vi "GUI_StagingEnergyCalib.vi"() -> ()   [LabVIEW 2013]
uses:
  Device Driver/StagingAnalysis/SubVis/SubVi/polTypDef.ctl
  Device Driver/StagingAnalysis/SubVis/energyCalibTypdef.ctl
  shared programs/GUI_Template/GUI_master/tcp new data cluster.ctl
  <vilib>/Analysis/1siggen.llb/Ramp Pattern by Samples.vi
  Device Driver/BaseDriver/BaseDriver.lvclass
  <vilib>/Analysis/NI_AALBase.lvlib
panel:
  out "Ramp Pattern":dbl[](graph)=[0.0, 4.5045045045045005e-06, 9.009009009009001e-06, 1.3513513513513502e-05, 1.8018018018018002e-05, 2.2522522522522503e-05, 2.7027027027027003e-05, 3.1531531531531504e-05, 3.6036036036036004e-05, 4.0540540540540505e-05, 4.5045045045045005e-05, 4.9549549549549506e-05, 5.4054054054054006e-05, 5.8558558558558507e-05, 6.306306306306301e-05, 6.756756756756751e-05, 7.207207207207201e-05, 7.657657657657652e-05, 8.108108108108101e-05, 8.558558558558552e-05, 9.009009009009001e-05, 9.459459459459452e-05, 9.909909909909901e-05, 0.00010360360360360352, 0.00010810810810810801, 0.00011261261261261252, 0.00011711711711711701, 0.00012162162162162152, 0.00012612612612612601, 0.00013063063063063052, 0.00013513513513513503, 0.0001396396396396395, 0.00014414414414414402, 0.00014864864864864852, 0.00015315315315315303, 0.0001576576576576575, 0.00016216216216216202, 0.00016666666666666653, 0.00017117117117117103, 0.00017567567567567554, 0.00018018018018018002, 0.00018468468468468453, 0.00018918918918918903, 0.00019369369369369354, 0.00019819819819819802, 0.00020270270270270253, 0.00020720720720720704, 0.00021171171171171154, 0.00021621621621621602, 0.00022072072072072053, 0.00022522522522522504, 0.00022972972972972955, 0.00023423423423423403, 0.00023873873873873853, 0.00024324324324324304, 0.00024774774774774755, 0.00025225225225225203, 0.00025675675675675656, 0.00026126126126126104, 0.0002657657657657655, 0.00027027027027027006, 0.00027477477477477454, 0.000279279279279279, 0.00028378378378378355, 0.00028828828828828803, 0.00029279279279279257, 0.00029729729729729705, 0.00030180180180180153, 0.00030630630630630606, 0.00031081081081081054, 0.000315315315315315, 0.00031981981981981956, 0.00032432432432432404, 0.00032882882882882857, 0.00033333333333333305, 0.00033783783783783753, 0.00034234234234234207, 0.00034684684684684655, 0.0003513513513513511, 0.00035585585585585556, 0.00036036036036036004, 0.0003648648648648646, 0.00036936936936936906, 0.00037387387387387354, 0.00037837837837837807, 0.00038288288288288255, 0.0003873873873873871, 0.00039189189189189156, 0.00039639639639639604, 0.0004009009009009006, 0.00040540540540540506, 0.00040990990990990954, 0.0004144144144144141, 0.00041891891891891855, 0.0004234234234234231, 0.00042792792792792757, 0.00043243243243243205, 0.0004369369369369366, 0.00044144144144144106, 0.00044594594594594554, 0.0004504504504504501, 0.00045495495495495456, 0.0004594594594594591, 0.00046396396396396357, 0.00046846846846846805, 0.0004729729729729726, 0.00047747747747747707, 0.00048198198198198155, 0.0004864864864864861, 0.0004909909909909906, 0.0004954954954954951, 0.0004999999999999996, 0.0005045045045045041, 0.0005090090090090085, 0.0005135135135135131, 0.0005180180180180176, 0.0005225225225225221, 0.0005270270270270266, 0.000531531531531531, 0.0005360360360360356, 0.0005405405405405401, 0.0005450450450450446, 0.0005495495495495491, 0.0005540540540540536, 0.000558558558558558, 0.0005630630630630626, 0.0005675675675675671, 0.0005720720720720716, 0.0005765765765765761, 0.0005810810810810805, 0.0005855855855855851, 0.0005900900900900896, 0.0005945945945945941, 0.0005990990990990986, 0.0006036036036036031, 0.0006081081081081076, 0.0006126126126126121, 0.0006171171171171166, 0.0006216216216216211, 0.0006261261261261256, 0.00063063063063063, 0.0006351351351351346, 0.0006396396396396391, 0.0006441441441441436, 0.0006486486486486481, 0.0006531531531531526, 0.0006576576576576571, 0.0006621621621621616, 0.0006666666666666661, 0.0006711711711711706, 0.0006756756756756751, 0.0006801801801801797, 0.0006846846846846841, 0.0006891891891891886, 0.0006936936936936931, 0.0006981981981981976, 0.0007027027027027022, 0.0007072072072072066, 0.0007117117117117111, 0.0007162162162162156, 0.0007207207207207201, 0.0007252252252252246, 0.0007297297297297292, 0.0007342342342342336, 0.0007387387387387381, 0.0007432432432432426, 0.0007477477477477471, 0.0007522522522522517, 0.0007567567567567561, 0.0007612612612612606, 0.0007657657657657651, 0.0007702702702702696, 0.0007747747747747742, 0.0007792792792792786, 0.0007837837837837831, 0.0007882882882882876, 0.0007927927927927921, 0.0007972972972972966, 0.0008018018018018012, 0.0008063063063063056, 0.0008108108108108101, 0.0008153153153153146, 0.0008198198198198191, 0.0008243243243243237, 0.0008288288288288281, 0.0008333333333333326, 0.0008378378378378371, 0.0008423423423423416, 0.0008468468468468462, 0.0008513513513513507, 0.0008558558558558551, 0.0008603603603603596, 0.0008648648648648641, 0.0008693693693693687, 0.0008738738738738732, 0.0008783783783783776, 0.0008828828828828821, 0.0008873873873873866, 0.0008918918918918911, 0.0008963963963963957, 0.0009009009009009002, 0.0009054054054054046, 0.0009099099099099091, 0.0009144144144144136, 0.0009189189189189182, 0.0009234234234234227, 0.0009279279279279271, 0.0009324324324324316, 0.0009369369369369361, 0.0009414414414414407, 0.0009459459459459452, 0.0009504504504504497, 0.0009549549549549541, 0.0009594594594594586, 0.0009639639639639631, 0.0009684684684684677, 0.0009729729729729722, 0.0009774774774774766, 0.0009819819819819812, 0.0009864864864864856, 0.0009909909909909902, 0.0009954954954954946, 0.0009999999999999992, 0.0010045045045045037, 0.0010090090090090081, 0.0010135135135135127, 0.001018018018018017, 0.0010225225225225217, 0.0010270270270270263, 0.0010315315315315306, 0.0010360360360360352, 0.0010405405405405396, 0.0010450450450450442, 0.0010495495495495488, 0.0010540540540540531, 0.0010585585585585577, 0.001063063063063062, 0.0010675675675675667, 0.0010720720720720713, 0.0010765765765765756, 0.0010810810810810802, 0.0010855855855855846, 0.0010900900900900892, 0.0010945945945945936, 0.0010990990990990982, 0.0011036036036036027, 0.0011081081081081071, 0.0011126126126126117, 0.001117117117117116, 0.0011216216216216207, 0.0011261261261261252, 0.0011306306306306296, 0.0011351351351351342, 0.0011396396396396386, 0.0011441441441441432, 0.0011486486486486478, 0.0011531531531531521, 0.0011576576576576567, 0.001162162162162161, 0.0011666666666666657, 0.0011711711711711703, 0.0011756756756756746, 0.0011801801801801792, 0.0011846846846846836, 0.0011891891891891882, 0.0011936936936936928, 0.0011981981981981971, 0.0012027027027027017, 0.0012072072072072061, 0.0012117117117117107, 0.0012162162162162153, 0.0012207207207207197, 0.0012252252252252242, 0.0012297297297297286, 0.0012342342342342332, 0.0012387387387387378, 0.0012432432432432422, 0.0012477477477477468, 0.0012522522522522511, 0.0012567567567567557, 0.00126126126126126, 0.0012657657657657647, 0.0012702702702702693, 0.0012747747747747736, 0.0012792792792792782, 0.0012837837837837826, 0.0012882882882882872, 0.0012927927927927918, 0.0012972972972972961, 0.0013018018018018007, 0.001306306306306305, 0.0013108108108108097, 0.0013153153153153143, 0.0013198198198198187, 0.0013243243243243232, 0.0013288288288288276, 0.0013333333333333322, 0.0013378378378378368, 0.0013423423423423412, 0.0013468468468468458, 0.0013513513513513501, 0.0013558558558558547, 0.0013603603603603593, 0.0013648648648648637, 0.0013693693693693683, 0.0013738738738738726, 0.0013783783783783772, 0.0013828828828828818, 0.0013873873873873862, 0.0013918918918918908, 0.0013963963963963951, 0.0014009009009008997, 0.0014054054054054043, 0.0014099099099099087, 0.0014144144144144133, 0.0014189189189189177, 0.0014234234234234222, 0.0014279279279279266, 0.0014324324324324312, 0.0014369369369369358, 0.0014414414414414402, 0.0014459459459459448, 0.0014504504504504491, 0.0014549549549549537, 0.0014594594594594583, 0.0014639639639639627, 0.0014684684684684673, 0.0014729729729729716, 0.0014774774774774762, 0.0014819819819819808, 0.0014864864864864852, 0.0014909909909909898, 0.0014954954954954941, 0.0014999999999999987, 0.0015045045045045033, 0.0015090090090090077, 0.0015135135135135123, 0.0015180180180180167, 0.0015225225225225212, 0.0015270270270270258, 0.0015315315315315302, 0.0015360360360360348, 0.0015405405405405392, 0.0015450450450450437, 0.0015495495495495483, 0.0015540540540540527, 0.0015585585585585573, 0.0015630630630630617, 0.0015675675675675663, 0.0015720720720720708, 0.0015765765765765752, 0.0015810810810810798, 0.0015855855855855842, 0.0015900900900900888, 0.0015945945945945931, 0.0015990990990990977, 0.0016036036036036023, 0.0016081081081081067, 0.0016126126126126113, 0.0016171171171171156, 0.0016216216216216202, 0.0016261261261261248, 0.0016306306306306292, 0.0016351351351351338, 0.0016396396396396382, 0.0016441441441441427, 0.0016486486486486473, 0.0016531531531531517, 0.0016576576576576563, 0.0016621621621621607, 0.0016666666666666653, 0.0016711711711711698, 0.0016756756756756742, 0.0016801801801801788, 0.0016846846846846832, 0.0016891891891891878, 0.0016936936936936924, 0.0016981981981981967, 0.0017027027027027013, 0.0017072072072072057, 0.0017117117117117103, 0.0017162162162162149, 0.0017207207207207192, 0.0017252252252252238, 0.0017297297297297282, 0.0017342342342342328, 0.0017387387387387374, 0.0017432432432432417, 0.0017477477477477463, 0.0017522522522522507, 0.0017567567567567553, 0.0017612612612612597, 0.0017657657657657643, 0.0017702702702702688, 0.0017747747747747732, 0.0017792792792792778, 0.0017837837837837822, 0.0017882882882882868, 0.0017927927927927914, 0.0017972972972972957, 0.0018018018018018003, 0.0018063063063063047, 0.0018108108108108093, 0.0018153153153153139, 0.0018198198198198182, 0.0018243243243243228, 0.0018288288288288272, 0.0018333333333333318, 0.0018378378378378364, 0.0018423423423423407, 0.0018468468468468453, 0.0018513513513513497, 0.0018558558558558543, 0.0018603603603603589, 0.0018648648648648633, 0.0018693693693693678, 0.0018738738738738722, 0.0018783783783783768, 0.0018828828828828814, 0.0018873873873873858, 0.0018918918918918903, 0.0018963963963963947, 0.0019009009009008993, 0.001905405405405404, 0.0019099099099099083, 0.0019144144144144129, 0.0019189189189189172, 0.0019234234234234218, 0.0019279279279279262, 0.0019324324324324308, 0.0019369369369369354, 0.0019414414414414397, 0.0019459459459459443, 0.0019504504504504487, 0.0019549549549549533, 0.0019594594594594577, 0.0019639639639639625, 0.001968468468468467, 0.001972972972972971, 0.001977477477477476, 0.0019819819819819804, 0.0019864864864864848, 0.001990990990990989, 0.001995495495495494, 0.0019999999999999983, 0.0020045045045045027, 0.0020090090090090075, 0.002013513513513512, 0.0020180180180180162, 0.0020225225225225206, 0.0020270270270270254, 0.0020315315315315298, 0.002036036036036034, 0.002040540540540539, 0.0020450450450450433, 0.0020495495495495477, 0.0020540540540540525, 0.002058558558558557, 0.0020630630630630612, 0.0020675675675675656, 0.0020720720720720704, 0.002076576576576575, 0.002081081081081079, 0.002085585585585584, 0.0020900900900900883, 0.0020945945945945927, 0.0020990990990990975, 0.002103603603603602, 0.0021081081081081063, 0.0021126126126126106, 0.0021171171171171154, 0.00212162162162162, 0.002126126126126124, 0.002130630630630629, 0.0021351351351351334, 0.0021396396396396377, 0.0021441441441441425, 0.002148648648648647, 0.0021531531531531513, 0.0021576576576576557, 0.0021621621621621605, 0.002166666666666665, 0.002171171171171169, 0.002175675675675674, 0.0021801801801801784, 0.0021846846846846828, 0.002189189189189187, 0.002193693693693692, 0.0021981981981981963, 0.0022027027027027007, 0.0022072072072072055, 0.00221171171171171, 0.0022162162162162142, 0.002220720720720719, 0.0022252252252252234, 0.0022297297297297278, 0.002234234234234232, 0.002238738738738737, 0.0022432432432432413, 0.0022477477477477457, 0.0022522522522522505, 0.002256756756756755, 0.0022612612612612592, 0.002265765765765764, 0.0022702702702702684, 0.002274774774774773, 0.002279279279279277, 0.002283783783783782, 0.0022882882882882863, 0.0022927927927927907, 0.0022972972972972955, 0.0023018018018018, 0.0023063063063063043, 0.002310810810810809, 0.0023153153153153134, 0.002319819819819818, 0.002324324324324322, 0.002328828828828827, 0.0023333333333333314, 0.0023378378378378357, 0.0023423423423423405, 0.002346846846846845, 0.0023513513513513493, 0.0023558558558558537, 0.0023603603603603585, 0.002364864864864863, 0.002369369369369367, 0.002373873873873872, 0.0023783783783783764, 0.0023828828828828807, 0.0023873873873873856, 0.00239189189189189, 0.0023963963963963943, 0.0024009009009008987, 0.0024054054054054035, 0.002409909909909908, 0.0024144144144144122, 0.002418918918918917, 0.0024234234234234214, 0.0024279279279279258, 0.0024324324324324306, 0.002436936936936935, 0.0024414414414414393, 0.0024459459459459437, 0.0024504504504504485, 0.002454954954954953, 0.0024594594594594572, 0.002463963963963962, 0.0024684684684684664, 0.002472972972972971, 0.0024774774774774756, 0.00248198198198198, 0.0024864864864864843, 0.0024909909909909887, 0.0024954954954954935, 0.002499999999999998, 0.0025045045045045023, 0.002509009009009007, 0.0025135135135135114, 0.002518018018018016, 0.00252252252252252, 0.002527027027027025, 0.0025315315315315294, 0.0025360360360360337, 0.0025405405405405385, 0.002545045045045043, 0.0025495495495495473, 0.002554054054054052, 0.0025585585585585565, 0.002563063063063061, 0.002567567567567565, 0.00257207207207207, 0.0025765765765765744, 0.0025810810810810787, 0.0025855855855855835, 0.002590090090090088, 0.0025945945945945923, 0.002599099099099097, 0.0026036036036036015, 0.002608108108108106, 0.00261261261261261, 0.002617117117117115, 0.0026216216216216194, 0.0026261261261261238, 0.0026306306306306286, 0.002635135135135133, 0.0026396396396396373, 0.002644144144144142, 0.0026486486486486465, 0.002653153153153151, 0.0026576576576576552, 0.00266216216216216, 0.0026666666666666644, 0.0026711711711711688, 0.0026756756756756736, 0.002680180180180178, 0.0026846846846846823, 0.0026891891891891867, 0.0026936936936936915, 0.002698198198198196, 0.0027027027027027003, 0.002707207207207205, 0.0027117117117117094, 0.002716216216216214, 0.0027207207207207186, 0.002725225225225223, 0.0027297297297297273, 0.0027342342342342317, 0.0027387387387387365, 0.002743243243243241, 0.0027477477477477453, 0.00275225225225225, 0.0027567567567567544, 0.002761261261261259, 0.0027657657657657636, 0.002770270270270268, 0.0027747747747747724, 0.0027792792792792767, 0.0027837837837837815, 0.002788288288288286, 0.0027927927927927903, 0.002797297297297295, 0.0028018018018017995, 0.002806306306306304, 0.0028108108108108086, 0.002815315315315313, 0.0028198198198198174, 0.0028243243243243218, 0.0028288288288288266, 0.002833333333333331, 0.0028378378378378353, 0.00284234234234234, 0.0028468468468468445, 0.002851351351351349, 0.0028558558558558532, 0.002860360360360358, 0.0028648648648648624, 0.0028693693693693668, 0.0028738738738738716, 0.002878378378378376, 0.0028828828828828803, 0.002887387387387385, 0.0028918918918918895, 0.002896396396396394, 0.0029009009009008982, 0.002905405405405403, 0.0029099099099099074, 0.002914414414414412, 0.0029189189189189166, 0.002923423423423421, 0.0029279279279279253, 0.00293243243243243, 0.0029369369369369345, 0.002941441441441439, 0.0029459459459459433, 0.002950450450450448, 0.0029549549549549524, 0.002959459459459457, 0.0029639639639639616, 0.002968468468468466, 0.0029729729729729704, 0.002977477477477475, 0.0029819819819819795, 0.002986486486486484, 0.0029909909909909883, 0.002995495495495493, 0.0029999999999999975, 0.003004504504504502, 0.0030090090090090066, 0.003013513513513511, 0.0030180180180180154, 0.0030225225225225198, 0.0030270270270270246, 0.003031531531531529, 0.0030360360360360333, 0.003040540540540538, 0.0030450450450450425, 0.003049549549549547, 0.0030540540540540517, 0.003058558558558556, 0.0030630630630630604, 0.0030675675675675648, 0.0030720720720720696, 0.003076576576576574, 0.0030810810810810783, 0.003085585585585583, 0.0030900900900900875, 0.003094594594594592, 0.0030990990990990967, 0.003103603603603601, 0.0031081081081081054, 0.00311261261261261, 0.0031171171171171146, 0.003121621621621619, 0.0031261261261261233, 0.003130630630630628, 0.0031351351351351325, 0.003139639639639637, 0.0031441441441441417, 0.003148648648648646, 0.0031531531531531504, 0.003157657657657655, 0.0031621621621621596, 0.003166666666666664, 0.0031711711711711684, 0.003175675675675673, 0.0031801801801801775, 0.003184684684684682, 0.0031891891891891863, 0.003193693693693691, 0.0031981981981981955, 0.0032027027027027, 0.0032072072072072046, 0.003211711711711709, 0.0032162162162162134, 0.003220720720720718, 0.0032252252252252226, 0.003229729729729727, 0.0032342342342342313, 0.003238738738738736, 0.0032432432432432405, 0.003247747747747745, 0.0032522522522522497, 0.003256756756756754, 0.0032612612612612584, 0.003265765765765763, 0.0032702702702702676, 0.003274774774774772, 0.0032792792792792763, 0.003283783783783781, 0.0032882882882882855, 0.00329279279279279, 0.0032972972972972947, 0.003301801801801799, 0.0033063063063063034, 0.0033108108108108082, 0.0033153153153153126, 0.003319819819819817, 0.0033243243243243213, 0.003328828828828826, 0.0033333333333333305, 0.003337837837837835, 0.0033423423423423397, 0.003346846846846844, 0.0033513513513513484, 0.003355855855855853, 0.0033603603603603576, 0.003364864864864862, 0.0033693693693693664, 0.003373873873873871, 0.0033783783783783755, 0.00338288288288288, 0.0033873873873873847, 0.003391891891891889, 0.0033963963963963935, 0.003400900900900898, 0.0034054054054054026, 0.003409909909909907, 0.0034144144144144114, 0.003418918918918916, 0.0034234234234234205, 0.003427927927927925, 0.0034324324324324297, 0.003436936936936934, 0.0034414414414414385, 0.003445945945945943, 0.0034504504504504476, 0.003454954954954952, 0.0034594594594594564, 0.003463963963963961, 0.0034684684684684656, 0.00347297297297297, 0.0034774774774774747, 0.003481981981981979, 0.0034864864864864835, 0.003490990990990988, 0.0034954954954954927, 0.003499999999999997, 0.0035045045045045014, 0.003509009009009006, 0.0035135135135135106, 0.003518018018018015, 0.0035225225225225193, 0.003527027027027024, 0.0035315315315315285, 0.003536036036036033, 0.0035405405405405377, 0.003545045045045042, 0.0035495495495495464, 0.0035540540540540512, 0.0035585585585585556, 0.00356306306306306, 0.0035675675675675643, 0.003572072072072069, 0.0035765765765765735, 0.003581081081081078, 0.0035855855855855827, 0.003590090090090087, 0.0035945945945945914, 0.0035990990990990963, 0.0036036036036036006, 0.003608108108108105, 0.0036126126126126094, 0.003617117117117114, 0.0036216216216216185, 0.003626126126126123, 0.0036306306306306277, 0.003635135135135132, 0.0036396396396396365, 0.0036441441441441413, 0.0036486486486486456, 0.00365315315315315, 0.0036576576576576544, 0.003662162162162159, 0.0036666666666666636, 0.003671171171171168, 0.0036756756756756727, 0.003680180180180177, 0.0036846846846846815, 0.003689189189189186, 0.0036936936936936907, 0.003698198198198195, 0.0037027027027026994, 0.003707207207207204, 0.0037117117117117086, 0.003716216216216213, 0.0037207207207207178, 0.003725225225225222, 0.0037297297297297265, 0.003734234234234231, 0.0037387387387387357, 0.00374324324324324, 0.0037477477477477444, 0.0037522522522522492, 0.0037567567567567536, 0.003761261261261258, 0.0037657657657657628, 0.003770270270270267, 0.0037747747747747715, 0.003779279279279276, 0.0037837837837837807, 0.003788288288288285, 0.0037927927927927894, 0.0037972972972972942, 0.0038018018018017986, 0.003806306306306303, 0.003810810810810808, 0.003815315315315312, 0.0038198198198198165, 0.003824324324324321, 0.0038288288288288257, 0.00383333333333333, 0.0038378378378378345, 0.0038423423423423393, 0.0038468468468468436, 0.003851351351351348, 0.0038558558558558524, 0.003860360360360357, 0.0038648648648648616, 0.003869369369369366, 0.0038738738738738707, 0.003878378378378375, 0.0038828828828828795, 0.0038873873873873843, 0.0038918918918918887, 0.003896396396396393, 0.0039009009009008974, 0.003905405405405402, 0.003909909909909907, 0.003914414414414411, 0.003918918918918915, 0.00392342342342342, 0.003927927927927925, 0.003932432432432429, 0.003936936936936934, 0.0039414414414414385, 0.003945945945945942, 0.003950450450450447, 0.003954954954954952, 0.003959459459459456, 0.003963963963963961, 0.003968468468468465, 0.0039729729729729695, 0.003977477477477474, 0.003981981981981978, 0.003986486486486483, 0.003990990990990988, 0.003995495495495492, 0.003999999999999997, 0.004004504504504501, 0.004009009009009005, 0.00401351351351351, 0.004018018018018015, 0.004022522522522519, 0.004027027027027024, 0.0040315315315315285, 0.0040360360360360325, 0.004040540540540537, 0.004045045045045041, 0.004049549549549546, 0.004054054054054051, 0.004058558558558555, 0.0040630630630630596, 0.004067567567567564, 0.004072072072072068, 0.004076576576576573, 0.004081081081081078, 0.004085585585585582, 0.004090090090090087, 0.0040945945945945915, 0.004099099099099095, 0.0041036036036036, 0.004108108108108105, 0.004112612612612609, 0.004117117117117114, 0.0041216216216216186, 0.0041261261261261225, 0.004130630630630627, 0.004135135135135131, 0.004139639639639636, 0.004144144144144141, 0.004148648648648645, 0.00415315315315315, 0.004157657657657654, 0.004162162162162158, 0.004166666666666663, 0.004171171171171168, 0.004175675675675672, 0.004180180180180177, 0.0041846846846846815, 0.004189189189189185, 0.00419369369369369, 0.004198198198198195, 0.004202702702702699, 0.004207207207207204, 0.004211711711711708, 0.0042162162162162125, 0.004220720720720717, 0.004225225225225221, 0.004229729729729726, 0.004234234234234231, 0.004238738738738735, 0.00424324324324324, 0.004247747747747744, 0.004252252252252248, 0.004256756756756753, 0.004261261261261258, 0.004265765765765762, 0.004270270270270267, 0.0042747747747747715, 0.0042792792792792755, 0.00428378378378378, 0.004288288288288285, 0.004292792792792789, 0.004297297297297294, 0.004301801801801798, 0.004306306306306303, 0.004310810810810807, 0.004315315315315311, 0.004319819819819816, 0.004324324324324321, 0.004328828828828825, 0.00433333333333333, 0.0043378378378378345, 0.004342342342342338, 0.004346846846846843, 0.004351351351351348, 0.004355855855855852, 0.004360360360360357, 0.004364864864864862, 0.0043693693693693655, 0.00437387387387387, 0.004378378378378374, 0.004382882882882879, 0.004387387387387384, 0.004391891891891888, 0.004396396396396393, 0.004400900900900897, 0.004405405405405401, 0.004409909909909906, 0.004414414414414411, 0.004418918918918915, 0.00442342342342342, 0.0044279279279279245, 0.0044324324324324284, 0.004436936936936933, 0.004441441441441438, 0.004445945945945942, 0.004450450450450447, 0.004454954954954952, 0.0044594594594594555, 0.00446396396396396, 0.004468468468468464, 0.004472972972972969, 0.004477477477477474, 0.004481981981981978, 0.004486486486486483, 0.0044909909909909874, 0.004495495495495491, 0.004499999999999996]
  in  "end":dbl=0.004499999999999996
  in  "file path (dialog if empty)":path=path "V:/Y2013/02-Feb/13_0207/analysis/s8.txt"
  in  "load":bool=TRUE
  in  "startlinear":dbl=0.000828
  out "x+1":dbl=188.0
  in  "old calib":bool=TRUE
  in  "take data":bool
  out "energyCalib":T1={"p-pol"={"Beam1"=0.585575, "Beam2"=0.414425, "Tele"=0.004938, "startLinear"=0.0007, "best fit parameters"={"0"=0.88643, "1"=-3261.333361, "2"=6330262.535463, "3"=-3978154912.425541}}, "s-pol"={"Beam1"=0.585575, "Beam2"=0.414424708329109, "Tele"=0.004938, "position for fit"=0.000828, "best fit parameters"={"0"=0.042645, "1"=208.033972, "2"=-303343.534936, "3"=170108367.568354}}, "B-CaveFilter"=0.165}
  in  "toDB":bool=TRUE
  in  "B-Cave-Filter (value)":dbl=0.165
  in  "BCaveFilterStatus":enum16{"B-Cave filter in", "B-Cave filter out"}(ring)=enum."B-Cave filter out"
  in  "Polarization":T2=enum."s-polarized"
  in  "fit":bool
  in  "reset":bool
  out "XY Graph":cluster{dbl[], dbl[]}[](graph)
  out "GUIdevice 1":string="StagingPXISlow"
  in  "Measurements.Analysis2::1":dbl=6.4710866e-05 caption="Energy in raw" min=0.0 max=0.0
  in  "Measurements.Analysis1::1":dbl=3.059521e-06 caption="Energy out raw" min=0.0 max=0.0
  out "device status::1":string="no scan"
  in  "stop":bool
  out "UDP error message":string
  in  "insert tag":bool=TRUE
  # "last calib:"
  # "V:\\Y2012\\12-Dec\\12_1213\\analysis\\s4.txt"
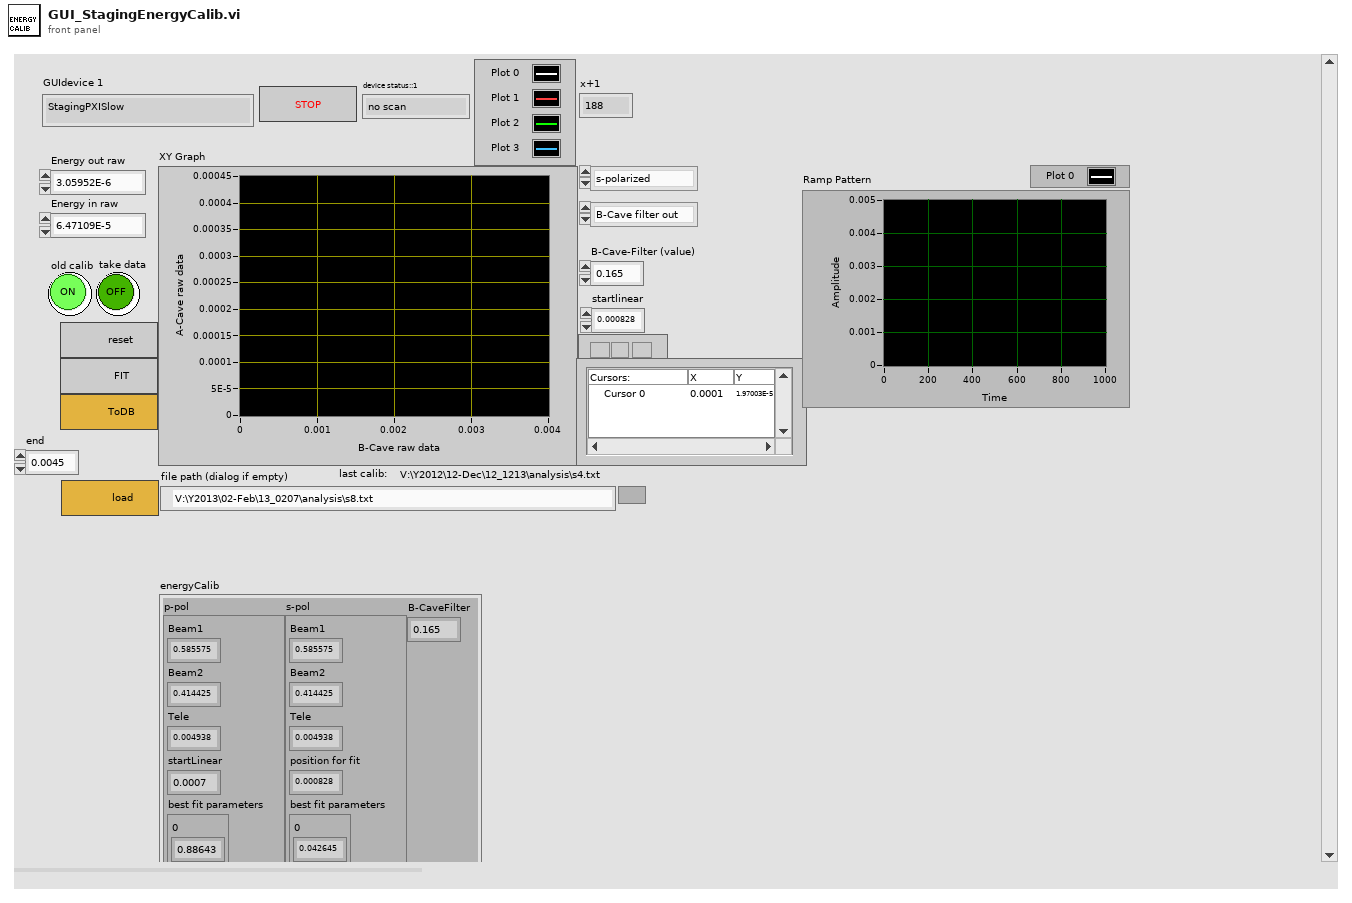
[diagram p1: front panel]
types:
  T1 = typedef "energyCalibTypdef.ctl" = cluster{"p-pol":cluster{"Beam1":dbl, "Beam2":dbl, "Tele":dbl, "startLinear":dbl, "best fit parameters":cluster{"0":dbl, "1":dbl, "2":dbl, "3":dbl}}, "s-pol":cluster{"Beam1":dbl, "Beam2":dbl, "Tele":dbl, "position for fit":dbl, "best fit parameters":cluster{"0":dbl, "1":dbl, "2":dbl, "3":dbl}}, "B-CaveFilter":dbl}
  T2 = typedef "polTypDef.ctl" = enum16{"p-polarized", "s-polarized"}
  T3 = typedef "tcp new data cluster.ctl" = cluster{"EventEnum":enum16{"new data", "connection status update"}, "Device name":string}
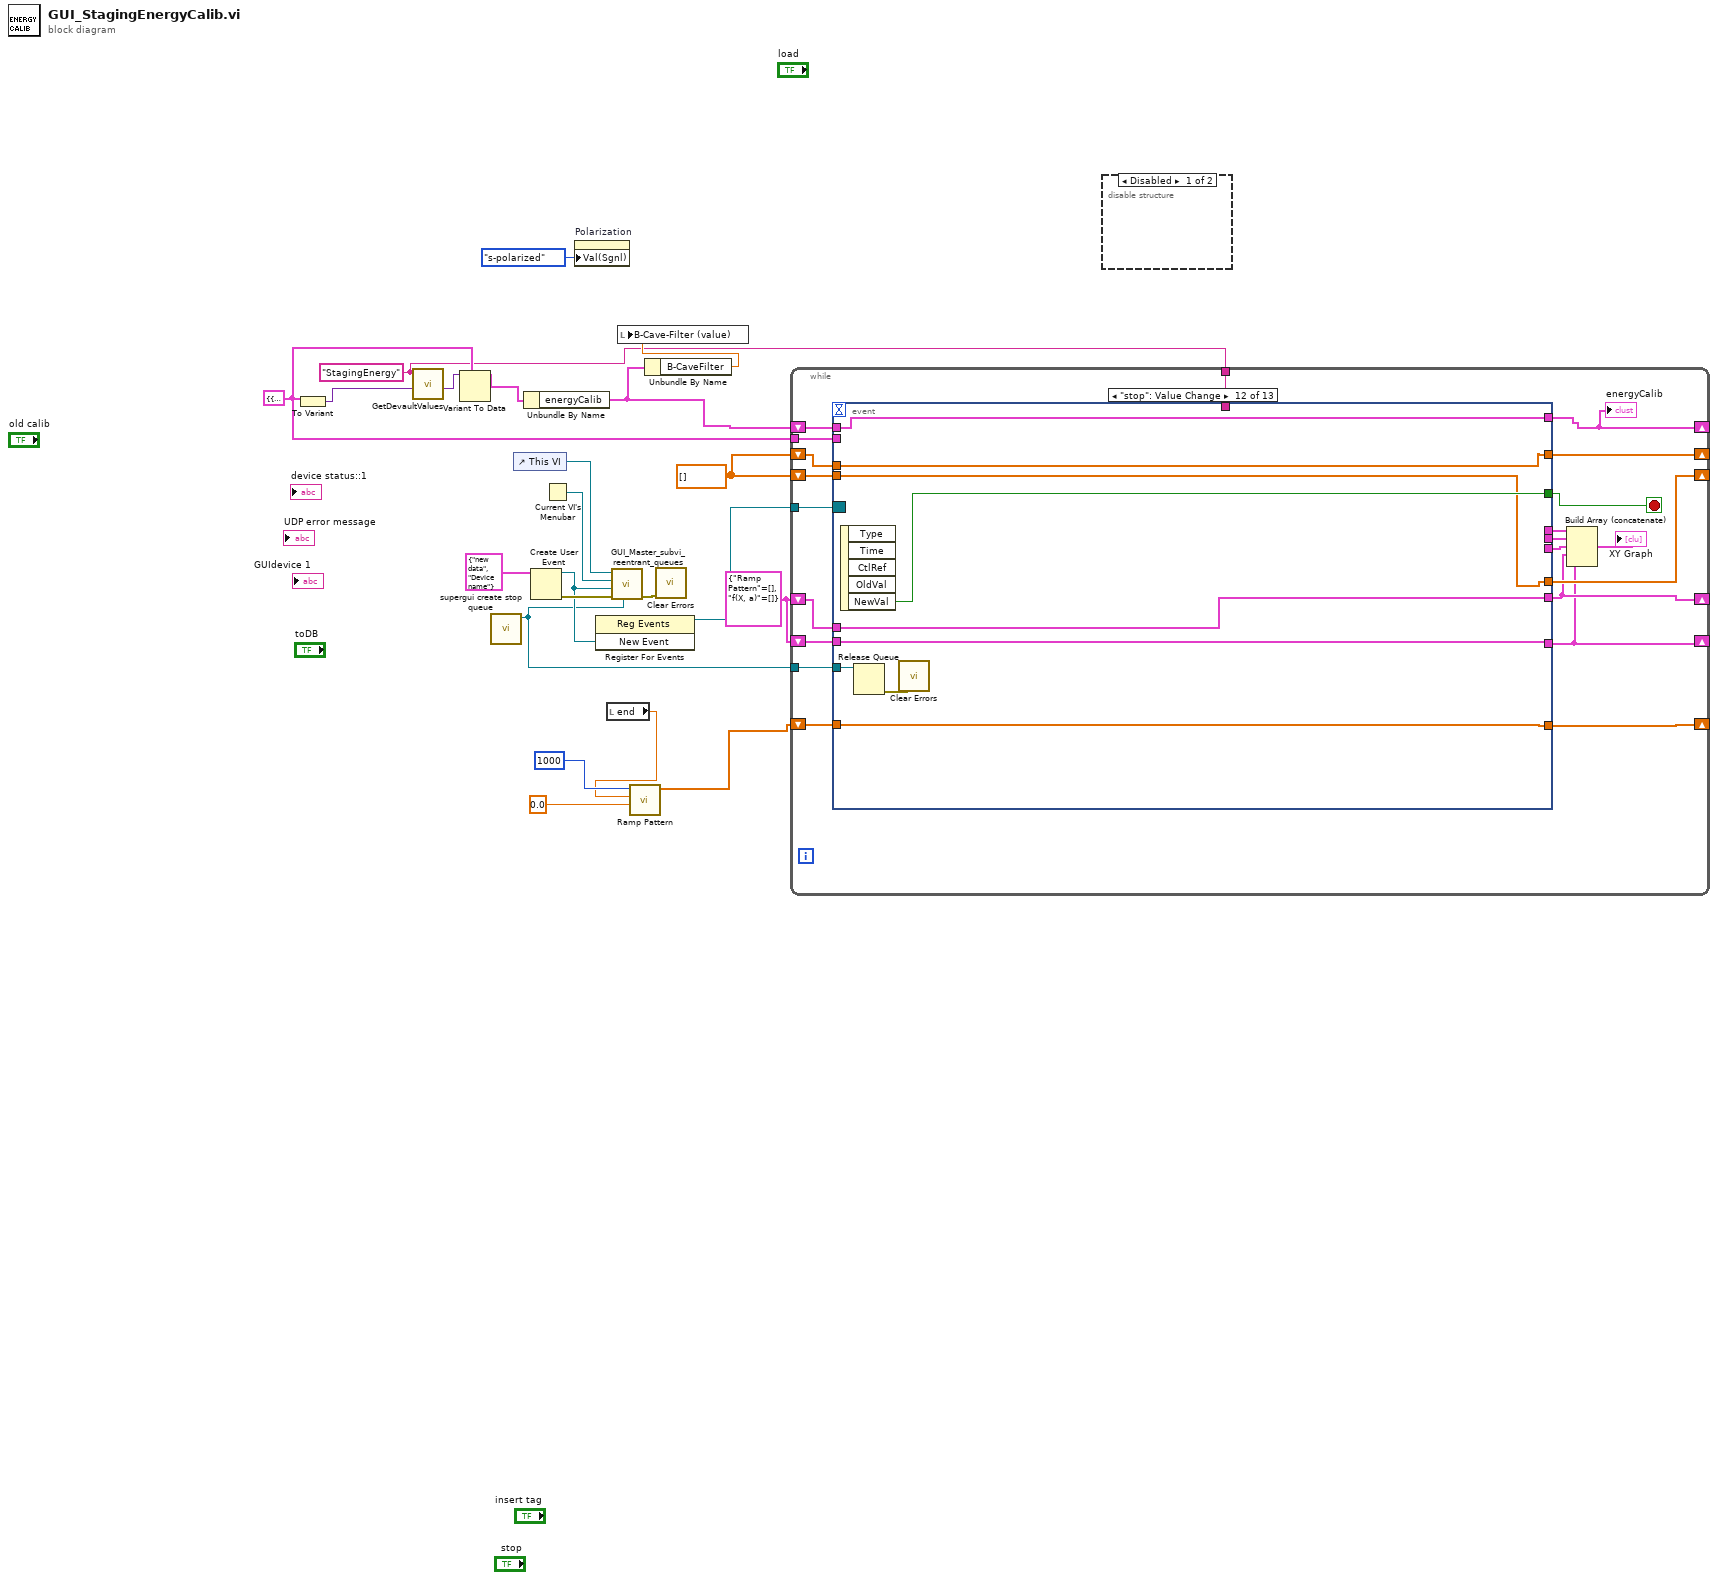
[diagram p0: block diagram]
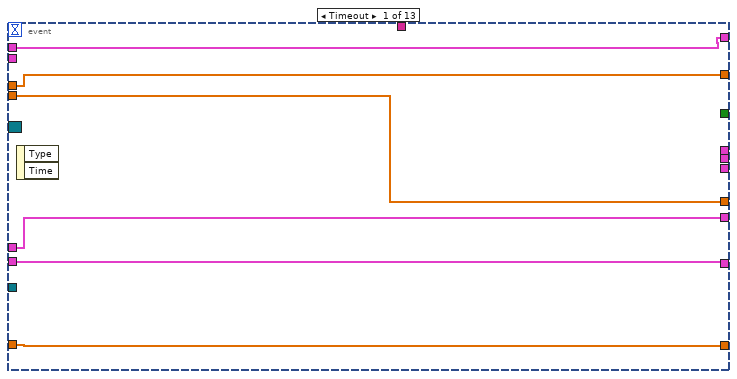
[diagram p3: hidden frame]
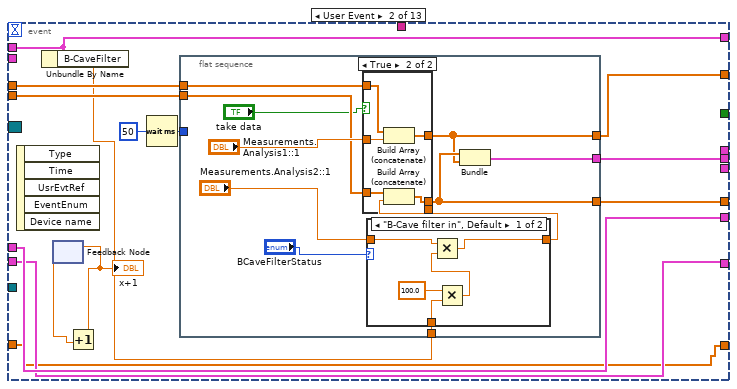
[diagram p4: hidden frame]
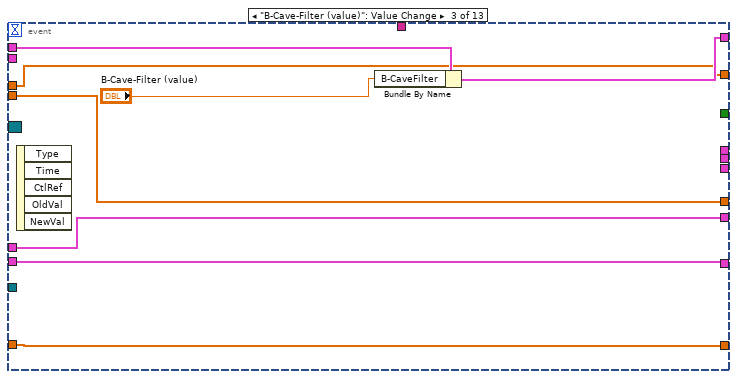
[diagram p7: hidden frame]
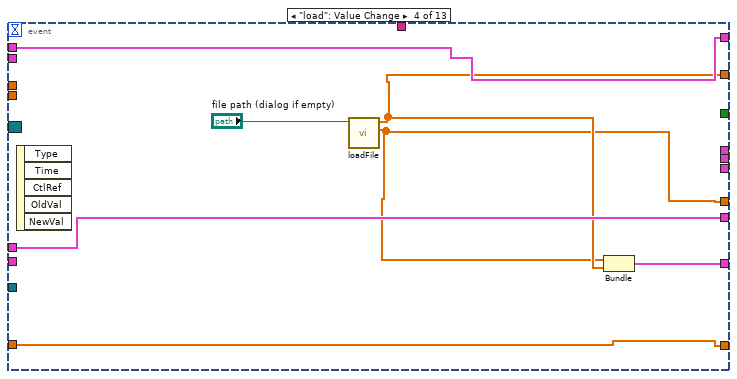
[diagram p8: hidden frame]
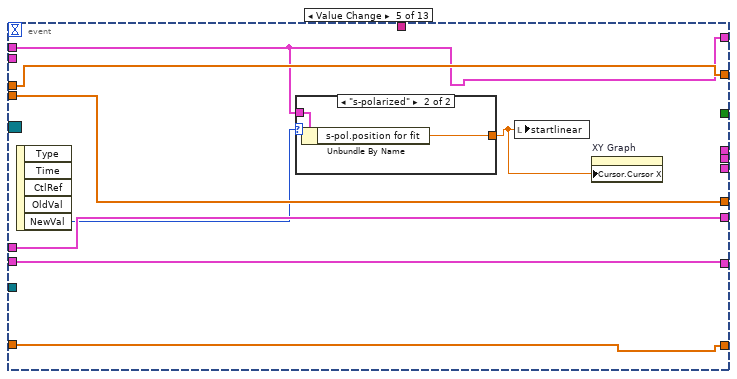
[diagram p9: hidden frame]
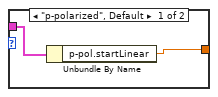
[diagram p10: hidden frame]
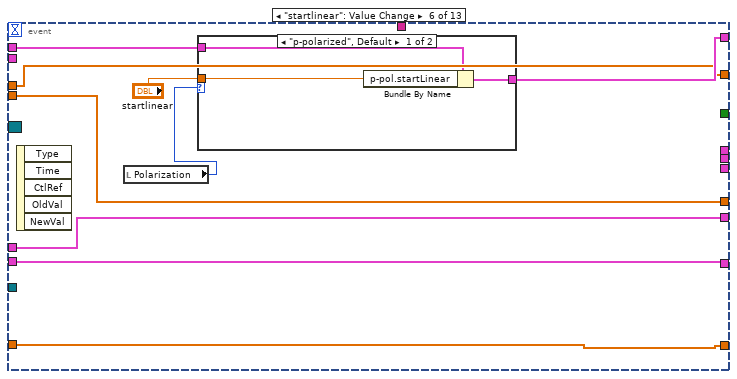
[diagram p11: hidden frame]
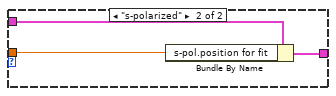
[diagram p12: hidden frame]
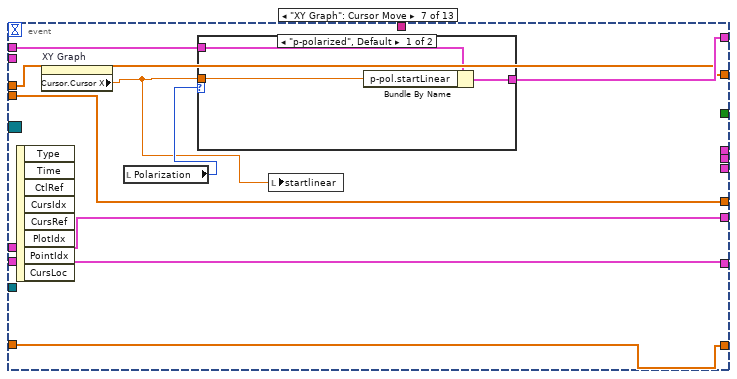
[diagram p13: hidden frame]
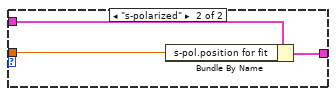
[diagram p14: hidden frame]
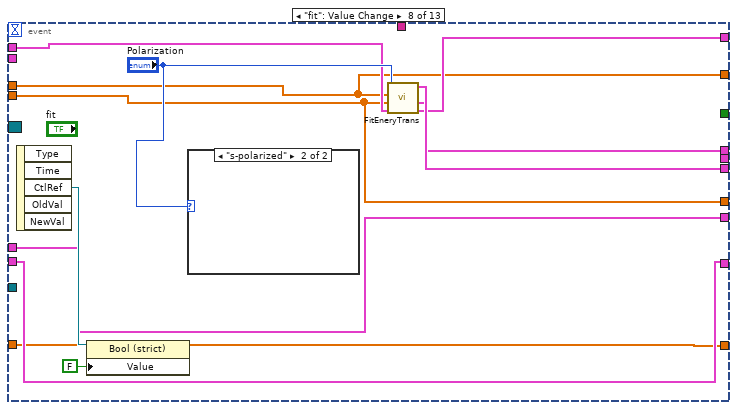
[diagram p15: hidden frame]
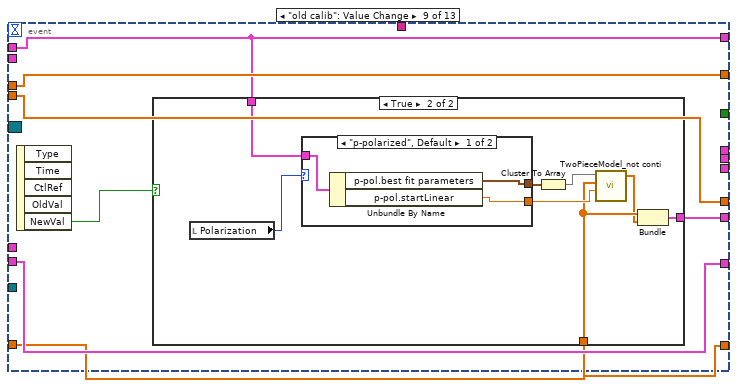
[diagram p17: hidden frame]
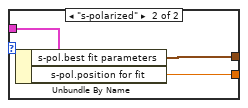
[diagram p19: hidden frame]
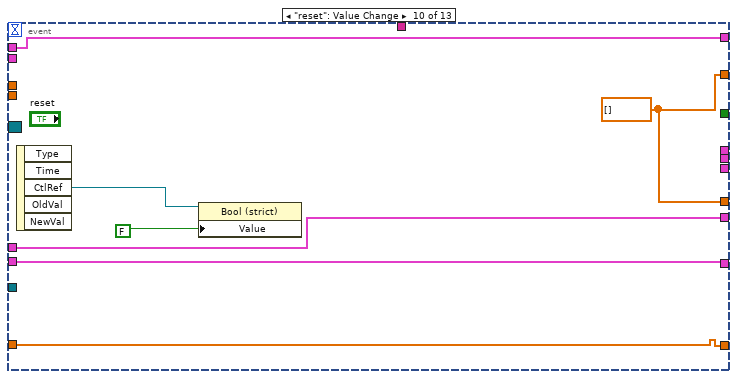
[diagram p20: hidden frame]
diagram:
  w6 = cluster{"Ramp Pattern":dbl[], "f(X, a)":dbl[]} {"Ramp Pattern"=[], "f(X, a)"=[]}
  w9 = cluster{"energyCalib":T1} {"energyCalib"={"p-pol"={"Beam1"=0.24495733496510103, "Beam2"=0.755042665034899, "Tele"=0.06901139685565201, "startLinear"=0.0007, "best fit parameters"={"0"=0.06577078607141854, "1"=1075.8816653301244, "2"=-1751262.2505806182, "3"=1069290462.0527091}}, "s-pol"={"Beam1"=0.5855752916708905, "Beam2"=0.4144247083291095, "Tele"=0.004937888283292143, "position for fit"=0.0007, "best fit parameters"={"0"=0.024167, "1"=188.618, "2"=-273128.0, "3"=156332000.0}}, "B-CaveFilter"=0.89}}
  w8 = "StagingEnergy" ("Device Name")
  w15 = dbl[] []
  n1 = To Variant(anything=w9) -> (Variant=w14:variant)
  n2 = call "GetDevaultValues.vi"("variant"=w14, "Device Name"=w8) -> ("variant out"=w13:variant)  [unwired: 7 in, 2 out]
  n3 = Variant To Data(type=w9, Variant=w13) -> (data=w12:cluster{"energyCalib":T1})  [unwired: 1 in, 1 out]
  n4 = call "supergui create stop queue.vi"() -> ("STOP Queue out"=w1:refnum<queue>)  [unwired: 11 in]
  n5 = control-ref of="This VI"() -> (w22:refnum<vi>)
  n6 = Unbundle By Name(w12) -> ("energyCalib"=w11:T1)
  n7 = Create User Event(user event datatype=T3 {"EventEnum"=enum."new data", "Device name"="Device name"} ("New Event")) -> (user event=w17:refnum<user-event>, error out=w19:errorcluster)  [unwired: 1 in]
  n8 = Current VI's Menubar() -> (w21:refnum<k9>)
  n9 = property on="Polarization" class="Enum (strict)"("Val(Sgnl)"=enum16{"p-polarized", "s-polarized"}."s-polarized" ("Value (Signaling)")) -> ()  [unwired: 2 in, 2 out]
  n10 = register-events(w17) -> (reference out=w16:refnum<event-registration>)  [unwired: 2 in, 1 out]
  n11 = local read "end"() -> (w3:dbl)
  n12 = call "GUI_Master_subvi_reentrant_queues.vi"("STOP Queue in"=w1, "error in (no error)"=w19, "tcp data event"=w17, "Caller menu reference"=w21, "Caller VI ref"=w22) -> ("error out"=w18:errorcluster)  [unwired: 6 in]
  n13 = call-poly <vilib>:"Ramp Pattern.vi"("start"=0.0, "end"=w3, "samples"=1000) -> ("Ramp Pattern"=w2:dbl[])  [unwired: 7 in, 1 out]
  n14 = Unbundle By Name(w11) -> ("B-CaveFilter"=w10:dbl)
  n15 = local write "B-Cave-Filter (value)"(w10) -> ()
  n16 = call <vilib>:"Clear Errors.vi"("error in (no error)"=w18) -> ()  [unwired: 6 in, 1 out]
  n17 = while {
    tunnel: w16 -> [w43]
    shift-right: [w41] -> _
    shift-left: w15 -> [w40]
    shift-right: [w39] -> _
    shift-left: w15 -> [w38]
    shift-right: [w30] -> _
    shift-left: w11 -> [w35]
    tunnel: w9 -> [w32]
    tunnel: w8 -> [w31]
    shift-right: [w28] -> _
    shift-left: w6 -> [w29]
    shift-right: [w26] -> _
    shift-left: w6 -> [w27]
    shift-right: [w25] -> _
    shift-left: w2 -> [w24]
    tunnel: w1 -> [w23]
    stop <- w42 stop-if-true
    n18 = event shown="[11] \"stop\": Value Change" {
      selector: w43 -> [_ _ _ _ _ _ _ _ _ _ _ _ _]
      dyn-events: _ -> [_ _ _ _ _ _ _ _ _ _ _ _ _]
      timeout: _ -> [_ _ _ _ _ _ _ _ _ _ _ _ _]
      tunnel: [_ _ _ _ _ _ _ _ _ _ _ w212 _] -> w42
      tunnel: [w49 w61 w93 w98 w111 w122 w137 w150 w164 w185 w196 w211 w221] -> w41
      tunnel: w40 -> [w49 w60 w93 _ w111 w122 w137 w150 w164 _ w196 w211 w221]
      tunnel: [w48 w59 w92 w97 w110 w121 w136 w149 w163 w185 w195 w210 w220] -> w39
      tunnel: w38 -> [w48 w58 w92 _ w110 w121 w136 w149 w163 _ w195 w210 w220]
      tunnel: [_ w57 _ _ _ _ _ _ _ _ _ _ _] -> w37
      tunnel: w35 -> [w47 w55 w96 w102 w107 w124 w139 w153 w162 w182 w193 w209 w219]
      tunnel: [_ _ _ _ _ _ _ w156 _ _ _ _ _] -> w34
      tunnel: [_ _ _ _ _ _ _ w152 _ _ _ _ _] -> w33
      tunnel: [w47 w55 w94 w102 w107 w123 w138 w151 w162 w182 w193 w209 w219] -> w30
      tunnel: w32 -> [_ _ _ _ _ _ _ _ _ _ w194 _ _]
      tunnel: w31 -> [_ _ _ _ _ _ _ _ _ _ w189 _ _]
      tunnel: [w46 w54 w91 w103 w109 w120 w135 w148 w161 w181 w188 w208 w218] -> w28
      tunnel: w29 -> [w46 w54 w91 w103 w109 w120 w135 w148 _ w181 w188 w208 w218]
      tunnel: [w45 w51 w90 w100 w105 w117 w132 w147 w159 w180 w187 w207 w217] -> w26
      tunnel: w27 -> [w45 w51 w90 _ w105 w117 w132 w147 w159 w180 w187 w207 w217]
      tunnel: [w44 w50 w89 w99 w104 w116 w131 w146 w158 w179 w186 w206 w213] -> w25
      tunnel: w24 -> [w44 w50 w89 w99 w104 w116 w131 w146 w158 w179 w186 w206 _]
      tunnel: w23 -> [_ _ _ _ _ _ _ _ _ _ _ w205 _]
      event Timeout {
        n19 = event-data() -> ()  [unwired: 1 in, 2 out]
      }
      event User Event {
        n20 = event-data() -> ()  [unwired: 1 in, 5 out]
        n21 = Unbundle By Name(w55) -> ("B-CaveFilter"=w56:dbl)
        n22 = feedback #1() -> (w52:dbl)  [unwired: 1 in]
        n23 = Increment(x=w52) -> (x+1=w53:dbl)
        "x+1" <- w53
        n24 = feedback-in #1(w53) -> ()
        n25 = Wait (ms)(milliseconds to wait=u32 50) -> (millisecond timer value=w62:u32)
        n26 = flat-sequence {
          tunnel: w62 -> [_]
          tunnel: [w64] -> w61
          tunnel: w60 -> [w73]
          tunnel: [w65] -> w59
          tunnel: w58 -> [w72]
          tunnel: [w71] -> w57
          tunnel: w56 -> [w67]
          frame #0 {
            n27 = case shown="\"B-Cave filter in\", Default" "BCaveFilterStatus" {
              tunnel: "Measurements.Analysis2::1" -> [w87 w88]
              tunnel: [w86 w88] -> w68
              tunnel: w67 -> [w85 _]
              frame "B-Cave filter in", Default {
                n28 = Multiply(x=100.0, y=w85) -> (x*y=w83:dbl)
                n29 = Multiply(x=w87, y=w83) -> (x*y=w86:dbl)
              }
              frame "B-Cave filter out" {
              }
            }
            n30 = case shown="True" "take data" {
              tunnel: "Measurements.Analysis1::1" -> [_ w82]
              tunnel: w73 -> [w76 w81]
              tunnel: w72 -> [w75 w80]
              tunnel: [w75 w79] -> w65
              tunnel: [w76 w78] -> w64
              tunnel: w68 -> [_ w77]
              frame False {
              }
              frame True {
                n31 = Build Array (concatenate)(w81, w82) -> (w78:dbl[])
                n32 = Build Array (concatenate)(w80, w77) -> (w79:dbl[])
              }
            }
            n33 = Bundle(w65, w64) -> (w71:cluster{dbl[], dbl[]})  [unwired: 1 in]
          }
        }
      }
      event "B-Cave-Filter (value)": Value Change {
        n34 = event-data() -> ()  [unwired: 1 in, 5 out]
        n35 = Bundle By Name(cluster=w96, "B-CaveFilter"="B-Cave-Filter (value)") -> (w94:T1)
      }
      event "load": Value Change {
        n36 = event-data() -> ()  [unwired: 1 in, 5 out]
        n37 = call "loadFile.vi"("file path (dialog if empty)"="file path (dialog if empty)") -> ("B-Cave"=w97:dbl[], "A-Cave"=w98:dbl[])  [unwired: 9 in]
        n38 = Bundle("B-Cave"=w97, "A-Cave"=w98) -> (w100:cluster{"B-Cave":dbl[], "A-Cave":dbl[]})  [unwired: 1 in]
      }
      event Value Change {
        n39 = event-data() -> ("NewVal"=w108:T2)  [unwired: 1 in, 4 out]
        n40 = case shown="\"s-polarized\"" w108 {
          tunnel: w107 -> [w113 w115]
          tunnel: [w112 w114] -> w106
          frame "p-polarized", Default {
            n41 = Unbundle By Name(w113) -> ("p-pol.startLinear"=w112:dbl)
          }
          frame "s-polarized" {
            n42 = Unbundle By Name(w115) -> ("s-pol.position for fit"=w114:dbl)
          }
        }
        n43 = local write "startlinear"(w106) -> ()
        n44 = property on="XY Graph" class="XYGraph (strict)"("Cursor.Cursor X"=w106) -> ()  [unwired: 2 in, 2 out]
      }
      event "startlinear": Value Change {
        n45 = event-data() -> ()  [unwired: 1 in, 5 out]
        n46 = local read "Polarization"() -> (w118:T2)
        n47 = case shown="\"p-polarized\", Default" w118 {
          tunnel: w124 -> [w127 w130]
          tunnel: [w126 w129] -> w123
          tunnel: "startlinear" -> [w125 w128]
          frame "p-polarized", Default {
            n48 = Bundle By Name(cluster=w127, "p-pol.startLinear"=w125) -> (w126:T1)
          }
          frame "s-polarized" {
            n49 = Bundle By Name(cluster=w130, "s-pol.position for fit"=w128) -> (w129:T1)
          }
        }
      }
      event "XY Graph": Cursor Move {
        n50 = event-data() -> ()  [unwired: 1 in, 8 out]
        n51 = property on="XY Graph" class="XYGraph (strict)"() -> ("Cursor.Cursor X"=w133:dbl)  [unwired: 2 in, 2 out]
        n52 = local read "Polarization"() -> (w134:T2)
        n53 = case shown="\"p-polarized\", Default" w134 {
          tunnel: w139 -> [w142 w145]
          tunnel: [w141 w144] -> w138
          tunnel: w133 -> [w140 w143]
          frame "p-polarized", Default {
            n54 = Bundle By Name(cluster=w142, "p-pol.startLinear"=w140) -> (w141:T1)
          }
          frame "s-polarized" {
            n55 = Bundle By Name(cluster=w145, "s-pol.position for fit"=w143) -> (w144:T1)
          }
        }
        n56 = local write "startlinear"(w133) -> ()
      }
      event "fit": Value Change {
        n57 = event-data() -> ("CtlRef"=w155:refnum<vi>)  [unwired: 1 in, 4 out]
        n58 = property class="Bool (strict)"(reference=w155, "Value"=FALSE) -> ()  [unwired: 1 in, 2 out]
        n59 = case shown="\"s-polarized\"" "Polarization" {
          frame "p-polarized", Default {
          }
          frame "s-polarized" {
          }
        }
        n60 = call "FitEneryTrans.vi"("energyCalib"=w153, "B-Cave Energy"=w149, "A-Cave Energy"=w150, "polarization"="Polarization") -> ("energyCalib out"=w151:T1, "transmission"=w152:cluster{"B-Cave Energy":dbl[], dbl[]}, "data and fit"=w156:cluster{"Array":dbl[], "Array 2":dbl[]}[])  [unwired: 4 in, 1 out]
      }
      event "old calib": Value Change {
        n61 = event-data() -> ("NewVal"=w160:bool)  [unwired: 1 in, 4 out]
        n62 = case shown="True" w160 {
          tunnel: w162 -> [_ w171]
          tunnel: w158 -> [_ w167]
          tunnel: [_ w165] -> w161
          frame False {
          }
          frame True {
            n63 = local read "Polarization"() -> (w172:T2)
            n64 = case shown="\"p-polarized\", Default" w172 {
              tunnel: w171 -> [w175 w178]
              tunnel: [w174 w177] -> w170
              tunnel: [w173 w176] -> w168
              frame "p-polarized", Default {
                n65 = Unbundle By Name(w175) -> ("p-pol.best fit parameters"=w174:cluster{"0":dbl, "1":dbl, "2":dbl, "3":dbl}, "p-pol.startLinear"=w173:dbl)
              }
              frame "s-polarized" {
                n66 = Unbundle By Name(w178) -> ("s-pol.best fit parameters"=w177:cluster{"0":dbl, "1":dbl, "2":dbl, "3":dbl}, "s-pol.position for fit"=w176:dbl)
              }
            }
            n67 = Cluster To Array(cluster=w170) -> (array=w169:dbl[])
            n68 = call "TwoPieceModel_not conti.vi"("data"=w168, "x"=w167, "a"=w169) -> ("f(X, a)"=w166:dbl[])  [unwired: 1 in, 2 out]
            n69 = Bundle("Ramp Pattern"=w167, "f(X, a)"=w166) -> (w165:cluster{"Ramp Pattern":dbl[], "f(X, a)":dbl[]})  [unwired: 1 in]
          }
        }
      }
      event "reset": Value Change {
        w185 = dbl[] []
        n70 = event-data() -> ("CtlRef"=w184:refnum<vi>)  [unwired: 1 in, 4 out]
        n71 = property class="Bool (strict)"(reference=w184, "Value"=FALSE) -> ()  [unwired: 1 in, 2 out]
      }
      event "toDB": Value Change {
        n72 = event-data() -> ()  [unwired: 1 in, 5 out]
        n73 = Bundle By Name(cluster=w194, "energyCalib"=w193) -> (w191:cluster{"energyCalib":T1})
        n74 = call "Get Cluster Element Names__ogtk_TS.vi"("Variant"=w191) -> ("Names (Array)"=w192:string[])  [unwired: 9 in, 1 out]
        n75 = To Variant(anything=w191) -> (Variant=w190:variant)
        n76 = for {
          tunnel: w192 -> [w202] mode=indexing
          tunnel: w190 -> [w203]
          tunnel: w189 -> [w197]
          n77 = call "Get Cluster Element by Name__ogtk_TS.vi"("Element Name"=w202, "Cluster"=w203) -> ("VElement"=w201:variant)  [unwired: 7 in, 2 out]
          n78 = Variant To Data(type=0.0, Variant=w201) -> (data=w199:dbl)  [unwired: 1 in, 1 out]
          n79 = Number To Fractional String(number=w199) -> (F-format string=w198:string)  [unwired: 3 in]
          n80 = call "UpdateVarDB.vi"("Value"=w198, "VarName"=w202, "Device Name"=w197) -> ()  [unwired: 8 in, 1 out]
        }
      }
      event "stop": Value Change {
        n81 = event-data() -> ("NewVal"=w212:bool)  [unwired: 1 in, 4 out]
        n82 = Release Queue(queue=w205) -> (error out=w204:errorcluster)  [unwired: 2 in, 2 out]
        n83 = call <vilib>:"Clear Errors.vi"("error in (no error)"=w204) -> ()  [unwired: 6 in, 1 out]
      }
      event "end": Value Change {
        n84 = event-data() -> ()  [unwired: 1 in, 5 out]
        n85 = call-poly <vilib>:"Ramp Pattern.vi"("start"=0.0, "end"="end", "samples"=1000) -> ("Ramp Pattern"=w213:dbl[])  [unwired: 7 in, 1 out]
        "Ramp Pattern" <- w213
      }
    }
    "energyCalib" <- w30
    n86 = Build Array (concatenate)(w33, w37, w34, w28, w26) -> (→"XY Graph":cluster{"Ramp Pattern":dbl[], "f(X, a)":dbl[]}[])
  }
  n87 = disable-structure shown="Disabled" {
    frame Disabled {
    }
    frame Enabled {
    }
  }
